vi "example.vi"() -> ()   [LabVIEW 2022 SP3, in "Cleaning cycle.lvclass"]
uses:
  Cleaning cycle.lvclass
panel:
  out "命令":cluster{"触发":bool, "周期项":T1}[](array[cluster])
  in  "简易流程周期设置":cluster{"switch button":bool, "设置按钮":bool}
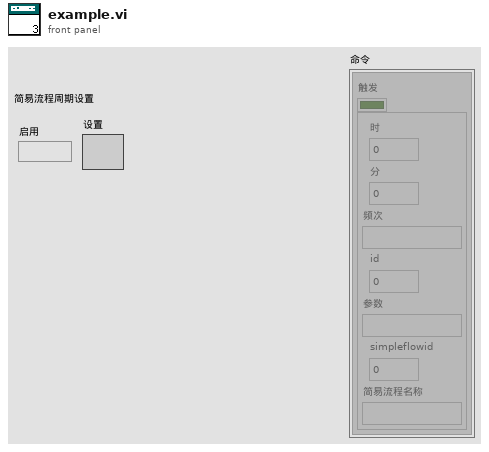
[diagram p1: front panel]
types:
  T1 = typedef "Cleaning cycle.lvclass/周期项.ctl" = cluster{"时":i32, "分":i32, "频次":string, "id":i32, "参数":string, "simpleflowid":i32, "简易流程名称":string}
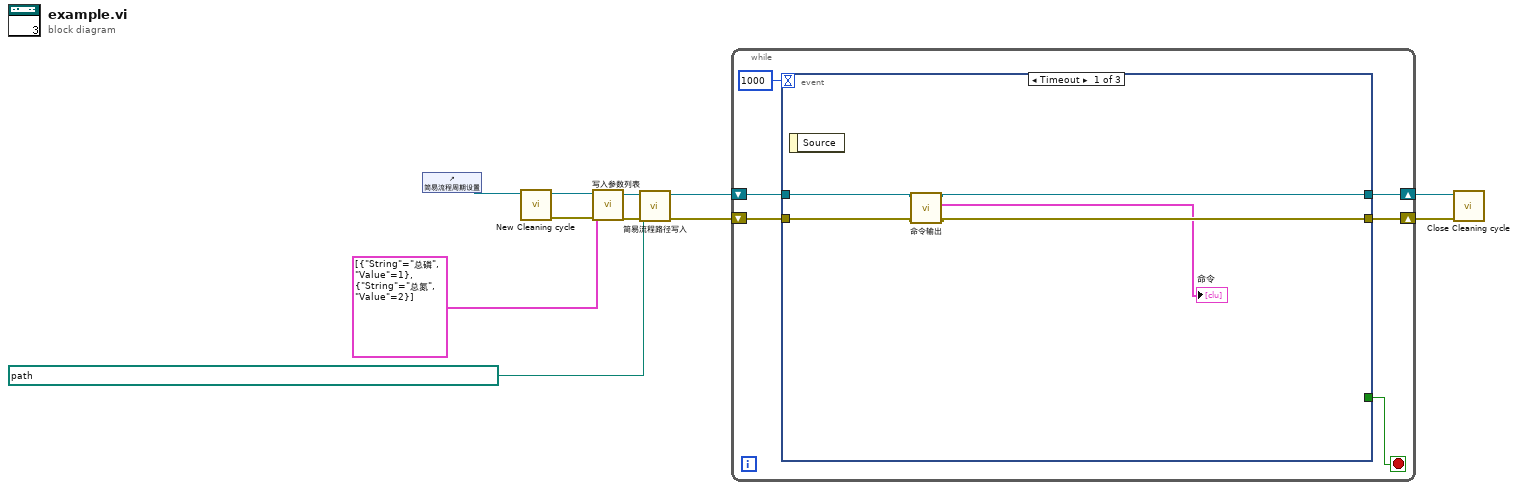
[diagram p0: block diagram]
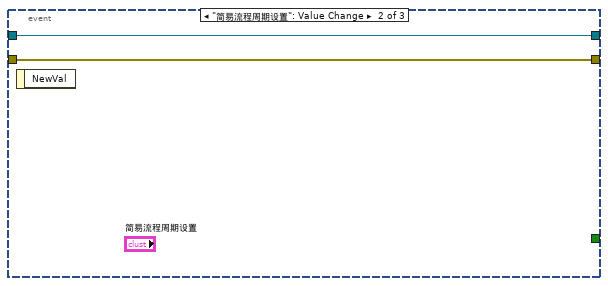
[diagram p2: hidden frame]
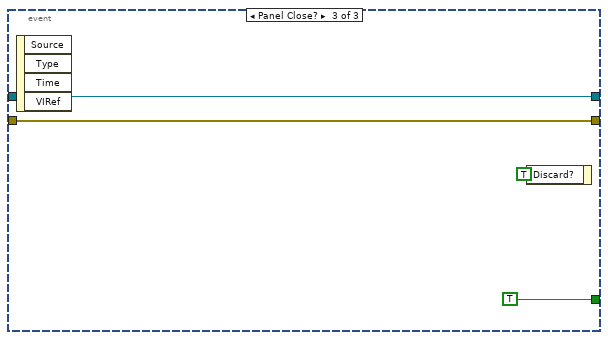
[diagram p3: hidden frame]
diagram:
  n1 = control-ref of="简易流程周期设置"() -> (w11:refnum<vi>)
  n2 = call "New Cleaning cycle.vi"("Reference"=w11) -> ("error out"=w3:errorcluster, "Cleaningcycle out"=w4:refnum<class "Cleaning cycle.lvclass">)  [unwired: 9 in]
  n3 = call "写入参数列表.vi"("error in (no error)"=w3, "参数列表"=cluster{"String":string, "Value":u16}[] [{"String"="总磷", "Value"=1}, {"String"="总氮", "Value"=2}], "Cleaningcycle 输入"=w4) -> ("error out"=w7:errorcluster, "Cleaningcycle 输出"=w8:refnum<class "Cleaning cycle.lvclass">)  [unwired: 7 in]
  n4 = call "简易流程路径写入.vi"("error in (no error)"=w7, "简易流程路径"=path "D:/Users/MCCP/Documents/新版软件流程文件夹/总磷总氮 复合步骤 20201202(1).xml", "Cleaningcycle 输入"=w8) -> ("error out"=w5:errorcluster, "Cleaningcycle 输出"=w6:refnum<class "Cleaning cycle.lvclass">)  [unwired: 7 in]
  n5 = while {
    shift-right: [w15] -> w10
    shift-left: w6 -> [w17]
    shift-right: [w14] -> w9
    shift-left: w5 -> [w16]
    stop <- w13 stop-if-true
    n6 = event shown="[0] Timeout" {
      selector: _ -> [_ _ _]
      dyn-events: _ -> [_ _ _]
      timeout: 1000 -> [_ _ _]
      tunnel: w17 -> [w22 w24 w28]
      tunnel: w16 -> [w21 w23 w27]
      tunnel: [w20 w24 w28] -> w15
      tunnel: [w19 w23 w27] -> w14
      tunnel: [_ _ TRUE] -> w13
      event Timeout {
        n7 = event-data() -> ()  [unwired: 1 in, 1 out]
        n8 = call "命令输出.vi"("error in (no error)"=w21, "Cleaningcycle 输入"=w22) -> ("error out"=w19:errorcluster, "命令"=→"命令":cluster{"触发":bool, "周期项":T1}[], "Cleaningcycle 输出"=w20:refnum<class "Cleaning cycle.lvclass">)  [unwired: 7 in]
      }
      event "简易流程周期设置": Value Change {
        n9 = event-data() -> ()  [unwired: 1 in, 1 out]
      }
      event Panel Close? {
        n10 = event-data() -> ()  [unwired: 1 in, 4 out]
        n11 = event-data("Discard?"=TRUE ("放弃？")) -> ()  [unwired: 1 in, 1 out]
      }
    }
  }
  n12 = call "Close Cleaning cycle.vi"("error in (no error)"=w9, "Cleaningcycle in"=w10) -> ()  [unwired: 9 in, 1 out]
